vi "QtoBeamDiameter.vi"(1 "wavelength":dbl, 2 "q":cdb) -> (0 "Beam diameter":dbl)   [LabVIEW 2011]
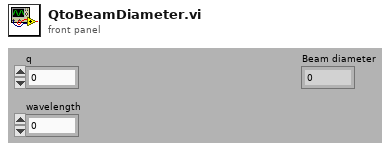
[diagram p1: front panel]
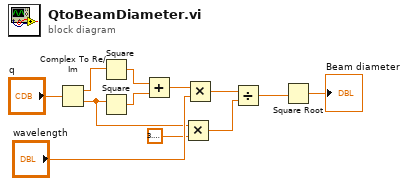
[diagram p0: block diagram]
diagram:
  n1 = Complex To Re/Im(x + iy="q") -> (x=w11:dbl, y=w5:dbl)
  n2 = Square(x=w11) -> (x^2=w10:dbl)
  n3 = Square(x=w5) -> (x^2=w9:dbl)
  n4 = Add(x=w10, y=w9) -> (x+y=w8:dbl)
  n5 = Multiply(x=w5, y=3.141592653589793) -> (x*y=w3:dbl)
  n6 = Multiply(x=w8, y="wavelength") -> (x*y=w4:dbl)
  n7 = Divide(x=w4, y=w3) -> (x/y=w2:dbl)
  n8 = Square Root(x=w2) -> (sqrt(x)=→"Beam diameter":dbl)
